vi "config file parser.vi"() -> ()   [LabVIEW 2011]
uses:
  PIDCluster.ctl
  <vilib>/Utility/file.llb/Read From Spreadsheet File (string).vi
  <vilib>/Rock Robotics/WPI/MotorControl/WPI_MotorControlOpen Jaguar.vi
  <vilib>/Rock Robotics/WPI/Solenoid/WPI_SolenoidOpenSingle.vi
panel:
  in  "path":string
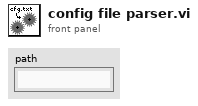
[diagram p1: front panel]
types:
  T1 = typedef "WPI_DigitalInputDevRef.ctl" = cluster{"DevStatus":errorcluster, "DIO Channel":T2, "Digital Module":T3}
  T2 = typedef "FPGA_DIOChannel.ctl" = enum8{"DIO 1", "DIO 2", "DIO 3", "DIO 4", "DIO 5", "DIO 6", "DIO 7", "DIO 8", "DIO 9", "DIO 10", "DIO 11", "DIO 12", "DIO 13", "DIO 14", "Invalid"}
  T3 = typedef "FPGA_TypedefDigitalModule.ctl" = enum16{"Digital Module 1", "Digital Module 2"}
  T4 = typedef "WPI_MotorControlDeviceRef.ctl" = cluster{"DeviceStatus":errorcluster, "Type":enum16{"PWM", "CAN"}, "PWM":cluster{"Digital Module":T3, "PWM Channel":T5, "DeadBand":T6}, "CAN":cluster{"Device Number":u8, "Control Mode":T7, "Semaphore":T8, "Max Vout":dbl}, "Invert":bool, "TransformRef":T9, "InvTransformRef":T9}
  T5 = typedef "FPGA_DIOPWMChannel.ctl" = enum8{"PWM 1", "PWM 2", "PWM 3", "PWM 4", "PWM 5", "PWM 6", "PWM 7", "PWM 8", "PWM 9", "PWM 10", "Invalid"}
  T6 = typedef "WPI_PWMDeadband.ctl" = cluster{"Name":string, "maxPositivePwm":i32, "minPositivePwm":i32, "centerPwm":i32, "maxNegativePwm":i32, "minNegativePwm":i32, "angularRange":u16}
  T7 = typedef "WPI_CANJaguar_ControlMode.ctl" = enum8{"Percent VBus", "Current", "Speed", "Position", "Voltage"}
  T8 = typedef "Semaphore RefNum" = refnum<k1>
  T9 = typedef "WPI_PWMTransform_ConPane.ctl" = refnum<vi>
  T10 = typedef "WPI_RelayDevRef.ctl" = cluster{"DevStatus":errorcluster, "Relay Channel":T11, "Digital Module":T3, "Relay Direction":T12}
  T11 = typedef "FPGA_DIORelayChannel.ctl" = enum8{"Relay 1", "Relay 2", "Relay 3", "Relay 4", "Relay 5", "Relay 6", "Relay 7", "Relay 8", "Invalid"}
  T12 = typedef "WPI_RelayDirection.ctl" = enum16{"Both directions", "Forward only", "Reverse only"}
  T13 = typedef "WPI_SolenoidDevRef.ctl" = cluster{"DevStatus":errorcluster, "Solenoid Module":T14, "Forward Solenoid Channel":T15, "Reverse Solenoid Channel":T15}
  T14 = typedef "FPGA_TypedefSolenoidModule.ctl" = enum16{"Solenoid Module 1", "Solenoid Module 2"}
  T15 = typedef "WPI_SolenoidChannel.ctl" = enum8{"Solenoid 1", "Solenoid 2", "Solenoid 3", "Solenoid 4", "Solenoid 5", "Solenoid 6", "Solenoid 7", "Solenoid 8", "Invalid"}
  T16 = typedef "PIDCluster.ctl" = cluster{"P":dbl, "I":dbl, "D":dbl}
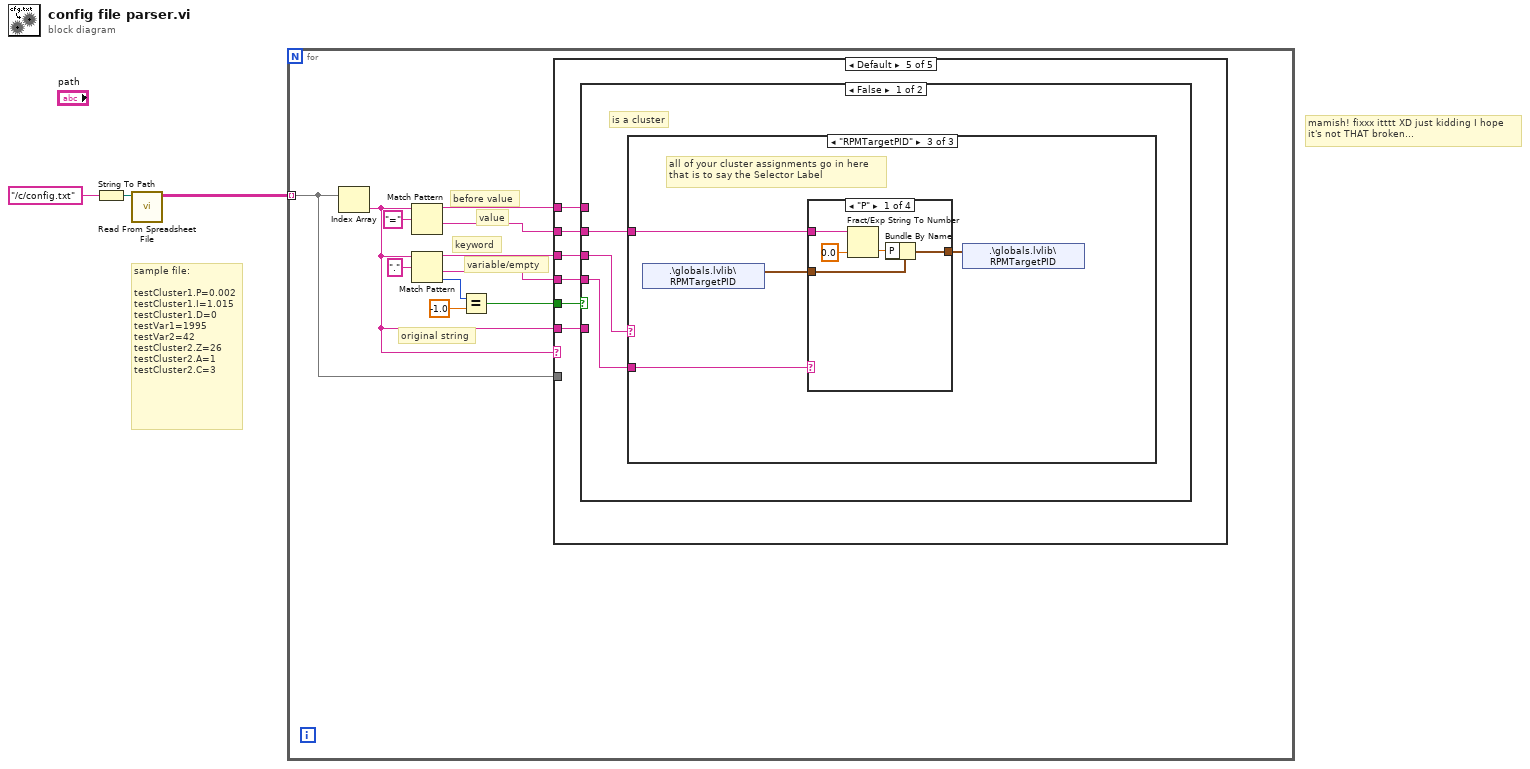
[diagram p0: block diagram]
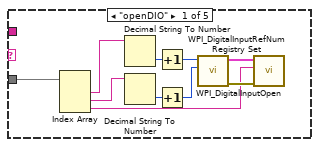
[diagram p2: hidden frame]
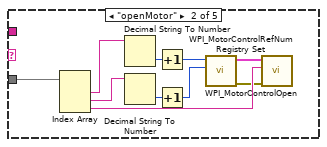
[diagram p3: hidden frame]
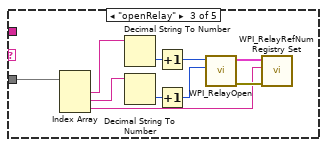
[diagram p4: hidden frame]
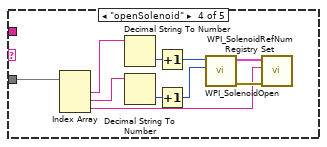
[diagram p5: hidden frame]
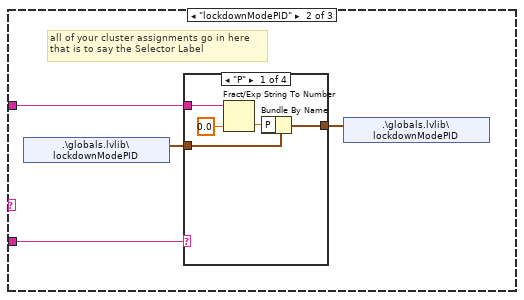
[diagram p7: hidden frame]
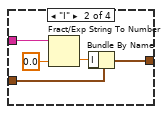
[diagram p8: hidden frame]
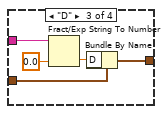
[diagram p9: hidden frame]
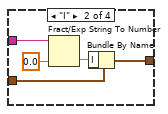
[diagram p11: hidden frame]
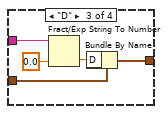
[diagram p12: hidden frame]
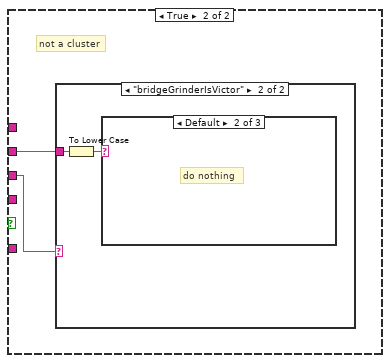
[diagram p14: hidden frame]
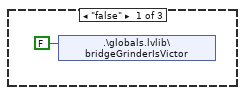
[diagram p16: hidden frame]
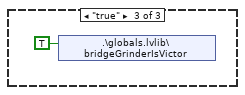
[diagram p17: hidden frame]
diagram:
  # "mamish! fixxx itttt XD just kidding I hope\nit's not THAT broken..."
  # "sample file:\n\ntestCluster1.P=0.002\ntestCluster1.I=1.015\ntestCluster1.D=0\ntestVar1=1995\ntestVar2=42\ntestCluster2.Z=26\ntestCluster2.A=1\ntestCluster2.C=3"
  n1 = String To Path(string="/c/config.txt") -> (path=w3:path)
  n2 = call-poly <vilib>:"Read From Spreadsheet File.vi"("file path (dialog if empty)"=w3) -> ("all rows"=w1:string[][])  [unwired: 6 in, 4 out]
  n3 = for {
    tunnel: w1 -> [w4] mode=indexing
    # "variable/empty"
    # "keyword"
    # "before value"
    # "value"
    # "original string"
    n4 = Index Array(array=w4) -> (element=w5:string)  [unwired: 1 in]
    n5 = Match Pattern(string=w5, regular expression="=") -> (before substring=w7:string, after substring=w8:string)  [unwired: 1 in, 2 out]
    n6 = Match Pattern(string=w5, regular expression=".") -> (before substring=w9:string, after substring=w6:string, offset past match=w11:i32)  [unwired: 1 in, 1 out]
    n7 = Equal?(x=w11, y=-1.0) -> (x = y?=w10:bool)
    n8 = case shown="Default" w5 {
      tunnel: w10 -> [_ _ _ _ w60]
      tunnel: w9 -> [_ _ _ _ w59]
      tunnel: w8 -> [_ _ _ _ w58]
      tunnel: w7 -> [_ _ _ _ w57]
      tunnel: w6 -> [_ _ _ _ w56]
      tunnel: w5 -> [_ _ _ _ w55]
      tunnel: w4 -> [w24 w28 w36 w46 _]
      frame "openDIO" {
        n9 = Index Array(array=w24) -> (element #1=w23:string, element #2=w22:string, element #3=w17:string)  [unwired: 3 in]
        n10 = Decimal String To Number(string=w23) -> (number=w21:i32)  [unwired: 2 in, 1 out]
        n11 = Decimal String To Number(string=w22) -> (number=w16:i32)  [unwired: 2 in, 1 out]
        n12 = Increment(x=w21) -> (x+1=w20:i32)
        n13 = Increment(x=w16) -> (x+1=w15:i32)
        n14 = call <vilib>:"WPI_DigitalInputOpen.vi"("DIO Channel"=w15, "Digital Module (Module 1)"=w20) -> ("error out"=w19:errorcluster, "DigitalInputDevRef"=w18:T1)  [unwired: 8 in]
        n15 = call <vilib>:"WPI_DigitalInputRefNum Registry Set.vi"("error in (no error)"=w19, "refnum name"=w17, "DigitalInputDevRef"=w18) -> ()  [unwired: 7 in, 2 out]
      }
      frame "openMotor" {
        n16 = Index Array(array=w28) -> (element #1=w29:string, element #2=w30:string, element #3=w34:string)  [unwired: 3 in]
        n17 = Decimal String To Number(string=w29) -> (number=w31:i32)  [unwired: 2 in, 1 out]
        n18 = Decimal String To Number(string=w30) -> (number=w26:i32)  [unwired: 2 in, 1 out]
        n19 = Increment(x=w31) -> (x+1=w32:i32)
        n20 = Increment(x=w26) -> (x+1=w25:i32)
        n21 = call-poly <vilib>:"WPI_MotorControlOpen.vi"("PWM Channel"=w25, "Digital Module (Module 1)"=w32) -> ("error out"=w33:errorcluster, "MotorControlDeviceRef"=w27:T4)  [unwired: 8 in]
        n22 = call <vilib>:"WPI_MotorControlRefNum Registry Set.vi"("error in (no error)"=w33, "refnum name"=w34, "MotorControlDevRef"=w27) -> ()  [unwired: 7 in, 2 out]
      }
      frame "openRelay" {
        n23 = Index Array(array=w36) -> (element #1=w42:string, element #2=w41:string, element #3=w37:string)  [unwired: 3 in]
        n24 = Decimal String To Number(string=w42) -> (number=w40:i32)  [unwired: 2 in, 1 out]
        n25 = Decimal String To Number(string=w41) -> (number=w43:i32)  [unwired: 2 in, 1 out]
        n26 = Increment(x=w40) -> (x+1=w39:i32)
        n27 = Increment(x=w43) -> (x+1=w44:i32)
        n28 = call <vilib>:"WPI_RelayOpen.vi"("Relay Channel"=w44, "Digital Module (Module 1)"=w39) -> ("error out"=w38:errorcluster, "RelayDevRef"=w35:T10)  [unwired: 8 in]
        n29 = call <vilib>:"WPI_RelayRefNum Registry Set.vi"("error in (no error)"=w38, "refnum name"=w37, "RelayDevRef"=w35) -> ()  [unwired: 7 in, 2 out]
      }
      frame "openSolenoid" {
        n30 = Index Array(array=w46) -> (element #1=w52:string, element #2=w51:string, element #3=w47:string)  [unwired: 3 in]
        n31 = Decimal String To Number(string=w52) -> (number=w50:i32)  [unwired: 2 in, 1 out]
        n32 = Decimal String To Number(string=w51) -> (number=w53:i32)  [unwired: 2 in, 1 out]
        n33 = Increment(x=w50) -> (x+1=w49:i32)
        n34 = Increment(x=w53) -> (x+1=w54:i32)
        n35 = call-poly <vilib>:"WPI_SolenoidOpen.vi"("Solenoid Channel"=w54, "Solenoid Module (Module 1)"=w49) -> ("error out"=w48:errorcluster, "SolenoidDevRef"=w45:T13)  [unwired: 8 in]
        n36 = call <vilib>:"WPI_SolenoidRefNum Registry Set.vi"("error in (no error)"=w48, "refnum name"=w47, "SolenoidDevRef"=w45) -> ()  [unwired: 7 in, 2 out]
      }
      frame Default {
        n37 = case shown="False" w60 {
          tunnel: w59 -> [w62 w105]
          tunnel: w58 -> [w63 w104]
          tunnel: w57 -> [_ _]
          tunnel: w56 -> [w61 _]
          tunnel: w55 -> [_ _]
          frame False {
            # "is a cluster"
            n38 = case shown="\"RPMTargetPID\"" w62 {
              tunnel: w63 -> [_ w66 w87]
              tunnel: w61 -> [_ w67 w85]
              frame Default {
                # "match not found, do nothing"
              }
              frame "lockdownModePID" {
                # "all of your cluster assignments go in here\nthat is to say the Selector Label"
                n39 = shared-variable ".\\globals.lvlib\\lockdownModePID"() -> (w65:T16)  [unwired: 1 in, 1 out]
                n40 = case shown="\"P\"" w67 {
                  tunnel: w66 -> [w71 w76 w80 _]
                  tunnel: w65 -> [w70 w75 w79 w83]
                  tunnel: [w69 w74 w78 w83] -> w64
                  frame "P" {
                    n41 = Fract/Exp String To Number(string=w71, default (0 dbl)=0.0 ("default (0 I32)")) -> (number=w68:dbl)  [unwired: 2 in, 1 out]
                    n42 = Bundle By Name(cluster=w70, "P"=w68) -> (w69:T16)
                  }
                  frame "I" {
                    n43 = Fract/Exp String To Number(string=w76, default (0 dbl)=0.0 ("default (0 I32)")) -> (number=w73:dbl)  [unwired: 2 in, 1 out]
                    n44 = Bundle By Name(cluster=w75, "I"=w73) -> (w74:T16)
                  }
                  frame "D" {
                    n45 = Fract/Exp String To Number(string=w80, default (0 dbl)=0.0 ("default (0 I32)")) -> (number=w81:dbl)  [unwired: 2 in, 1 out]
                    n46 = Bundle By Name(cluster=w79, "D"=w81) -> (w78:T16)
                  }
                  frame Default {
                    # "not found: do nothing"
                  }
                }
                n47 = shared-variable ".\\globals.lvlib\\lockdownModePID"(w64) -> ()  [unwired: 1 in, 1 out]
              }
              frame "RPMTargetPID" {
                # "all of your cluster assignments go in here\nthat is to say the Selector Label"
                n48 = shared-variable ".\\globals.lvlib\\RPMTargetPID"() -> (w86:T16)  [unwired: 1 in, 1 out]
                n49 = case shown="\"P\"" w85 {
                  tunnel: w87 -> [w91 w96 w100 _]
                  tunnel: w86 -> [w90 w95 w99 w103]
                  tunnel: [w89 w94 w98 w103] -> w84
                  frame "P" {
                    n50 = Fract/Exp String To Number(string=w91, default (0 dbl)=0.0 ("default (0 I32)")) -> (number=w88:dbl)  [unwired: 2 in, 1 out]
                    n51 = Bundle By Name(cluster=w90, "P"=w88) -> (w89:T16)
                  }
                  frame "I" {
                    n52 = Fract/Exp String To Number(string=w96, default (0 dbl)=0.0 ("default (0 I32)")) -> (number=w93:dbl)  [unwired: 2 in, 1 out]
                    n53 = Bundle By Name(cluster=w95, "I"=w93) -> (w94:T16)
                  }
                  frame "D" {
                    n54 = Fract/Exp String To Number(string=w100, default (0 dbl)=0.0 ("default (0 I32)")) -> (number=w101:dbl)  [unwired: 2 in, 1 out]
                    n55 = Bundle By Name(cluster=w99, "D"=w101) -> (w98:T16)
                  }
                  frame Default {
                    # "not found: do nothing"
                  }
                }
                n56 = shared-variable ".\\globals.lvlib\\RPMTargetPID"(w84) -> ()  [unwired: 1 in, 1 out]
              }
            }
          }
          frame True {
            # "not a cluster"
            n57 = case shown="\"bridgeGrinderIsVictor\"" w105 {
              tunnel: w104 -> [_ w107]
              frame Default {
                # "match not found, do nothing"
              }
              frame "bridgeGrinderIsVictor" {
                n58 = To Lower Case(string=w107) -> (all lower case string=w106:string)
                n59 = case shown="Default" w106 {
                  frame "false" {
                    n60 = shared-variable ".\\globals.lvlib\\bridgeGrinderIsVictor"(FALSE ("bridgeGrinderIsVictor")) -> ()  [unwired: 1 in, 1 out]
                  }
                  frame Default {
                    # "do nothing"
                  }
                  frame "true" {
                    n61 = shared-variable ".\\globals.lvlib\\bridgeGrinderIsVictor"(TRUE ("bridgeGrinderIsVictor")) -> ()  [unwired: 1 in, 1 out]
                  }
                }
              }
            }
          }
        }
      }
    }
  }
